vi "ex_5.vi"() -> ()   [LabVIEW 2020]
uses:
  #typedef_Student.ctl
panel:
  out "Array 2":i32[](array[numeric])
  out "Array":string[](array[string])
  out "sorted array":T1[](array[typedef])
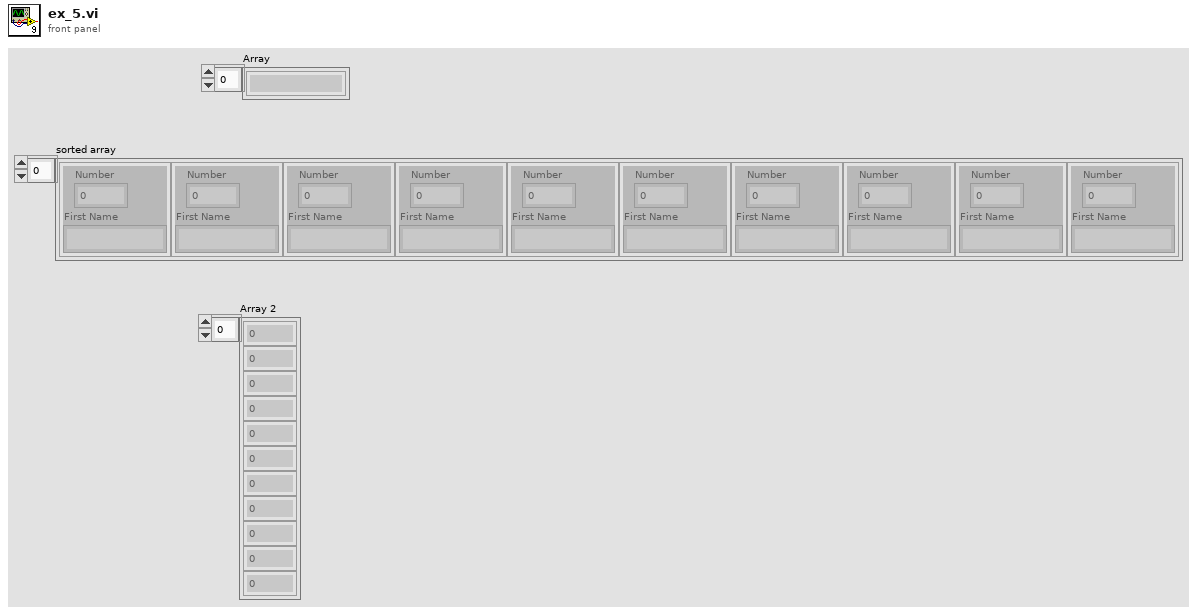
[diagram p1: front panel]
types:
  T1 = typedef "#typedef_Student.ctl" = cluster{"Number":i32, "First Name":string}
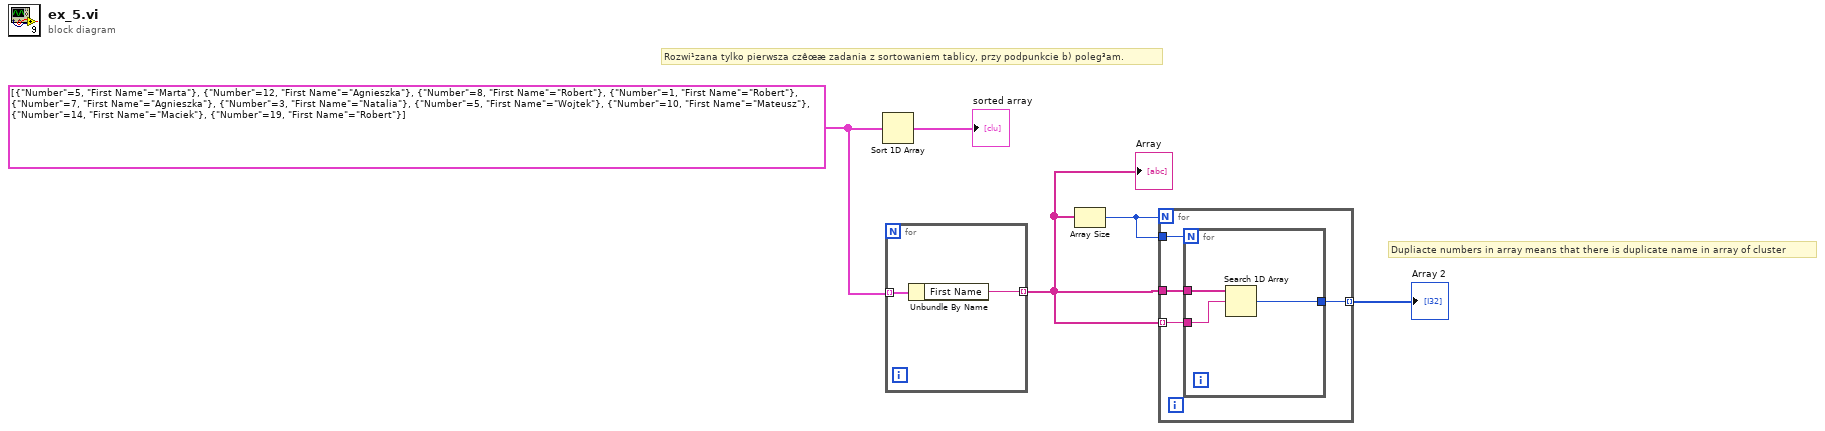
[diagram p0: block diagram]
diagram:
  w4 = T1[] [{"Number"=5, "First Name"="Marta"}, {"Number"=12, "First Name"="Agnieszka"}, {"Number"=8, "First Name"="Robert"}, {"Number"=1, "First Name"="Robert"}, {"Number"=7, "First Name"="Agnieszka"}, {"Number"=3, "First Name"="Natalia"}, {"Number"=5, "First Name"="Wojtek"}, {"Number"=10, "First Name"="Mateusz"}, {"Number"=14, "First Name"="Maciek"}, {"Number"=19, "First Name"="Robert"}]
  # "Rozwi¹zana tylko pierwsza czêœæ zadania z sortowaniem tablicy, przy podpunkcie b) poleg³am."
  # "Dupliacte numbers in array means that there is duplicate name in array of cluster"
  n1 = Sort 1D Array(array=w4) -> (sorted array=→"sorted array":T1[])
  n2 = for {
    tunnel: w4 -> [w7] mode=indexing
    tunnel: [w6] -> w2 mode=indexing
    n3 = Unbundle By Name(w7) -> ("First Name"=w6:string)
  }
  "Array" <- w2
  n4 = Array Size(array=w2) -> (size(s)=w1:i32)
  n5 = for {
    N: w1 -> [_]
    tunnel: w2 -> [w11] mode=indexing
    tunnel: [w10] -> w3 mode=indexing
    tunnel: w2 -> [w9]
    tunnel: w1 -> [w8]
    n6 = for {
      N: w8 -> [_]
      tunnel: w11 -> [w14]
      tunnel: [w13] -> w10
      tunnel: w9 -> [w12]
      n7 = Search 1D Array(1D array=w12, element=w14) -> (index of element=w13:i32)  [unwired: 1 in]
    }
  }
  "Array 2" <- w3
